vi "test_Study.vi"() -> ()   [LabVIEW 2023]
uses:
  Study/Study Actor/Study Actor/Study Actor.lvclass
  C:/Program Files/National Instruments/LabVIEW 2023/vi.lib/MGI/Panel Manager/Panel Actor/Panel Actor/Panel Actor.lvclass
  <vilib>/ni/Actors/Network Endpoint Actors/Protocols/Network Stream Strategy/Network Stream/Network Stream.lvclass/Network Stream.ctl
  <vilib>/ni/Actors/Network Endpoint Actors/Protocols/Network Stream Strategy/Network Stream Initiator/Network Stream Initiator.lvclass/Network Stream Initiator.ctl
  Study/Study Actor/Study Actor/Study Actor.lvclass/Study Actor.ctl
  <vilib>/ni/Actors/Network Endpoint Actors/Protocols/Network Stream Strategy/Network Stream/Write Buffer Size.vi
  <vilib>/ni/Actors/Network Endpoint Actors/Protocols/Network Stream Strategy/Network Stream/Write Name.vi
  <vilib>/ni/Actors/Network Endpoint Actors/Protocols/Network Stream Strategy/Network Stream Initiator/Network Stream Initiator.lvclass
  C:/Program Files/National Instruments/LabVIEW 2023/vi.lib/ni/Actors/Network Endpoint Actors/Protocols/Network Stream Strategy/Network Stream/Network Stream.lvclass
  C:/Program Files/National Instruments/LabVIEW 2023/vi.lib/ni/Actors/Network Endpoint Actors/Abstract Classes/Message Stream/Message Stream.lvclass
  <vilib>/MGI/Panel Manager/Panel/Window Position/Reference Position/Ref Top Level/Ref Top Level.lvclass
  C:/Program Files/National Instruments/LabVIEW 2023/vi.lib/MGI/Panel Manager/Panel/Window Position/Window Position.lvclass
  <vilib>/ni/Actors/Network Endpoint Actors/Protocols/Network Stream Strategy/Network Stream/Write Address.vi
  <vilib>/MGI/Panel Manager/Panel Actor/Panel Actor/Launch Root Panel Window.vi
  <vilib>/MGI/Panel Manager/Panel/Window Position/Reference Position/Ref Top Level/Ref Top Level.vi
  <vilib>/MGI/Panel Manager/Panel Actor/Panel Actor/Panel Actor.lvclass
  <vilib>/MGI/Panel Manager/Panel/Panel.lvlib
  C:/Program Files/National Instruments/LabVIEW 2023/vi.lib/MGI/Panel Manager/Panel/Window Position/Reference Position/Reference Position.lvclass
  C:/Program Files/National Instruments/LabVIEW 2023/vi.lib/MGI/Panel Manager/Panel/Window Position/Reference Position/Ref Top Level/Ref Top Level.lvclass
  C:/Program Files/National Instruments/LabVIEW 2023/vi.lib/ActorFramework/Actor/Actor.lvclass
  D:/git/HAL/HAL GOOP4/Study/Study Actor/Study Actor/Study Actor.lvclass
  D:/git/HAL/HAL GOOP4/Study/Study Actor/IStudy Actor/IStudy Actor.lvclass
  C:/Program Files/National Instruments/LabVIEW 2023/vi.lib/ni/Actors/Network Endpoint Actors/Nested Endpoint Caller/Nested Endpoint Caller/Nested Endpoint Caller.lvclass
panel:
  out "error out":errorcluster
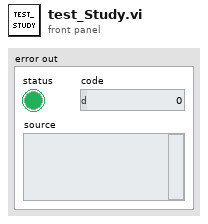
[diagram p1: front panel]
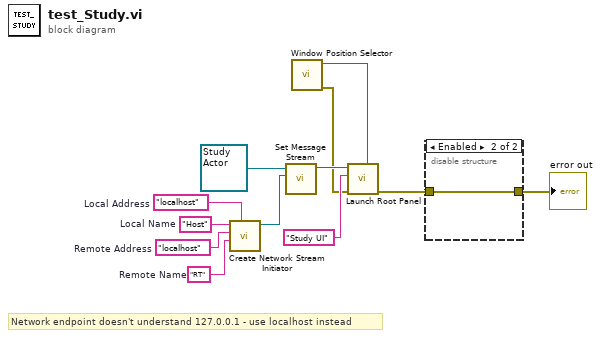
[diagram p0: block diagram]
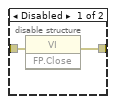
[diagram p2: hidden frame]
diagram:
  w8 = "RT"  # Remote Name
  w7 = "localhost"  # Local Address
  w9 = "localhost"  # Remote Address
  w10 = "Host"  # Local Name
  # "Network endpoint doesn't understand 127.0.0.1 - use localhost instead"
  n1 = call <vilib>:"Create Network Stream Initiator.vi"("Local Address"=w7, "Remote Name"=w8, "Remote Address"=w9, "Name"=w10) -> ("Network Stream Initiator out"=w5:refnum<class "Network Stream Initiator.lvclass">)  [unwired: 7 in]
  n2 = call "Set Message Stream.vi"("Message Stream.lvclass"=w5, "Study Actor in"=refnum<class "Study Actor.lvclass"> refnum ("HAL GOOP4.lvlib:Study Actor.lvlib:Study Actor.lvclass")) -> ("Study Actor out"=w6:refnum<class "Study Actor.lvclass">)  [unwired: 9 in]
  n3 = call-poly <vilib>:"Window Position Selector.vi"() -> ("Error Out"=w1:errorcluster, "Ref Top Level out"=w12:refnum<class "Ref Top Level.lvclass">)  [unwired: 10 in]
  n4 = call-poly <vilib>:"Launch Root Panel.vi"("Window Position (Maximize First Call)"=w12, "Error In"=w1, "Title"="Study UI", "Panel Actor in"=w6) -> ("Error Out"=w2:errorcluster)  [unwired: 6 in, 1 out]
  n5 = disable-structure shown="Enabled" {
    disable-tunnel: [w14 w15] -> w4
    disable-tunnel: w2 -> [w13 w15]
    frame Disabled {
      n6 = invoke class="VI" method="FP.Close"(error in=w13) -> (error out=w14:errorcluster)  [unwired: 2 in, 2 out]
    }
    frame Enabled {
    }
  }
  "error out" <- w4
